vi "数字量输入配置.vi"() -> ()   [LabVIEW 2010] (continued)
              n1455 = local write "单选_第47路"(w57) -> ()
              n1456 = local write "单选_第48路"(w57) -> ()
              n1457 = local write "单选_第49路"(w57) -> ()
              n1458 = local write "单选_第50路"(w57) -> ()
              n1459 = local write "单选_第51路"(w57) -> ()
              n1460 = local write "单选_第52路"(w57) -> ()
              n1461 = local write "单选_第53路"(w57) -> ()
              n1462 = local write "单选_第54路"(w57) -> ()
              n1463 = local write "单选_第55路"(w57) -> ()
              n1464 = local write "单选_第56路"(w57) -> ()
              n1465 = local write "单选_第57路"(w57) -> ()
              n1466 = local write "单选_第58路"(w57) -> ()
              n1467 = local write "单选_第59路"(w57) -> ()
              n1468 = local write "单选_第60路"(w57) -> ()
              n1469 = local write "单选_第61路"(w57) -> ()
              n1470 = local write "单选_第62路"(w57) -> ()
              n1471 = local write "单选_第63路"(w57) -> ()
              n1472 = local write "单选_第64路"(w57) -> ()
              n1473 = local write "单选_第71路"(w57) -> ()
              n1474 = local write "单选_第79路"(w57) -> ()
              n1475 = local write "单选_第65路"(w57) -> ()
              n1476 = local write "单选_第66路"(w57) -> ()
              n1477 = local write "单选_第67路"(w57) -> ()
              n1478 = local write "单选_第68路"(w57) -> ()
              n1479 = local write "单选_第69路"(w57) -> ()
              n1480 = local write "单选_第70路"(w57) -> ()
              n1481 = local write "单选_第72路"(w57) -> ()
              n1482 = local write "单选_第73路"(w57) -> ()
              n1483 = local write "单选_第74路"(w57) -> ()
              n1484 = local write "单选_第75路"(w57) -> ()
              n1485 = local write "单选_第76路"(w57) -> ()
              n1486 = local write "单选_第77路"(w57) -> ()
              n1487 = local write "单选_第78路"(w57) -> ()
              n1488 = local write "单选_第80路"(w57) -> ()
            }
            frame 13 {
              w58 = TRUE
              w59 = FALSE ("单选_第41路")
              n1489 = local write "单选_第1路"(w58) -> ()
              n1490 = local write "单选_第2路"(w58) -> ()
              n1491 = local write "单选_第3路"(w58) -> ()
              n1492 = local write "单选_第4路"(w58) -> ()
              n1493 = local write "单选_第5路"(w58) -> ()
              n1494 = local write "单选_第6路"(w58) -> ()
              n1495 = local write "单选_第7路"(w58) -> ()
              n1496 = local write "单选_第8路"(w58) -> ()
              n1497 = local write "单选_第9路"(w58) -> ()
              n1498 = local write "单选_第10路"(w58) -> ()
              n1499 = local write "单选_第11路"(w58) -> ()
              n1500 = local write "单选_第12路"(w58) -> ()
              n1501 = local write "单选_第13路"(w58) -> ()
              n1502 = local write "单选_第14路"(w59) -> ()
              n1503 = local write "单选_第15路"(w59) -> ()
              n1504 = local write "单选_第16路"(w59) -> ()
              n1505 = local write "单选_第17路"(w59) -> ()
              n1506 = local write "单选_第18路"(w59) -> ()
              n1507 = local write "单选_第19路"(w59) -> ()
              n1508 = local write "单选_第20路"(w59) -> ()
              n1509 = local write "单选_第21路"(w59) -> ()
              n1510 = local write "单选_第22路"(w59) -> ()
              n1511 = local write "单选_第23路"(w59) -> ()
              n1512 = local write "单选_第24路"(w59) -> ()
              n1513 = local write "单选_第25路"(w59) -> ()
              n1514 = local write "单选_第26路"(w59) -> ()
              n1515 = local write "单选_第27路"(w59) -> ()
              n1516 = local write "单选_第28路"(w59) -> ()
              n1517 = local write "单选_第29路"(w59) -> ()
              n1518 = local write "单选_第30路"(w59) -> ()
              n1519 = local write "单选_第31路"(w59) -> ()
              n1520 = local write "单选_第32路"(w59) -> ()
              n1521 = local write "单选_第33路"(w59) -> ()
              n1522 = local write "单选_第34路"(w59) -> ()
              n1523 = local write "单选_第35路"(w59) -> ()
              n1524 = local write "单选_第36路"(w59) -> ()
              n1525 = local write "单选_第37路"(w59) -> ()
              n1526 = local write "单选_第38路"(w59) -> ()
              n1527 = local write "单选_第39路"(w59) -> ()
              n1528 = local write "单选_第40路"(w59) -> ()
              n1529 = local write "单选_第41路"(w59) -> ()
              n1530 = local write "单选_第42路"(w59) -> ()
              n1531 = local write "单选_第43路"(w59) -> ()
              n1532 = local write "单选_第44路"(w59) -> ()
              n1533 = local write "单选_第45路"(w59) -> ()
              n1534 = local write "单选_第46路"(w59) -> ()
              n1535 = local write "单选_第47路"(w59) -> ()
              n1536 = local write "单选_第48路"(w59) -> ()
              n1537 = local write "单选_第49路"(w59) -> ()
              n1538 = local write "单选_第50路"(w59) -> ()
              n1539 = local write "单选_第51路"(w59) -> ()
              n1540 = local write "单选_第52路"(w59) -> ()
              n1541 = local write "单选_第53路"(w59) -> ()
              n1542 = local write "单选_第54路"(w59) -> ()
              n1543 = local write "单选_第55路"(w59) -> ()
              n1544 = local write "单选_第56路"(w59) -> ()
              n1545 = local write "单选_第57路"(w59) -> ()
              n1546 = local write "单选_第58路"(w59) -> ()
              n1547 = local write "单选_第59路"(w59) -> ()
              n1548 = local write "单选_第60路"(w59) -> ()
              n1549 = local write "单选_第61路"(w59) -> ()
              n1550 = local write "单选_第62路"(w59) -> ()
              n1551 = local write "单选_第63路"(w59) -> ()
              n1552 = local write "单选_第64路"(w59) -> ()
              n1553 = local write "单选_第71路"(w59) -> ()
              n1554 = local write "单选_第79路"(w59) -> ()
              n1555 = local write "单选_第65路"(w59) -> ()
              n1556 = local write "单选_第66路"(w59) -> ()
              n1557 = local write "单选_第67路"(w59) -> ()
              n1558 = local write "单选_第68路"(w59) -> ()
              n1559 = local write "单选_第69路"(w59) -> ()
              n1560 = local write "单选_第70路"(w59) -> ()
              n1561 = local write "单选_第72路"(w59) -> ()
              n1562 = local write "单选_第73路"(w59) -> ()
              n1563 = local write "单选_第74路"(w59) -> ()
              n1564 = local write "单选_第75路"(w59) -> ()
              n1565 = local write "单选_第76路"(w59) -> ()
              n1566 = local write "单选_第77路"(w59) -> ()
              n1567 = local write "单选_第78路"(w59) -> ()
              n1568 = local write "单选_第80路"(w59) -> ()
            }
            frame 14 {
              w60 = TRUE
              w61 = FALSE ("单选_第41路")
              n1569 = local write "单选_第1路"(w60) -> ()
              n1570 = local write "单选_第2路"(w60) -> ()
              n1571 = local write "单选_第3路"(w60) -> ()
              n1572 = local write "单选_第4路"(w60) -> ()
              n1573 = local write "单选_第5路"(w60) -> ()
              n1574 = local write "单选_第6路"(w60) -> ()
              n1575 = local write "单选_第7路"(w60) -> ()
              n1576 = local write "单选_第8路"(w60) -> ()
              n1577 = local write "单选_第9路"(w60) -> ()
              n1578 = local write "单选_第10路"(w60) -> ()
              n1579 = local write "单选_第11路"(w60) -> ()
              n1580 = local write "单选_第12路"(w60) -> ()
              n1581 = local write "单选_第13路"(w60) -> ()
              n1582 = local write "单选_第14路"(w60) -> ()
              n1583 = local write "单选_第15路"(w61) -> ()
              n1584 = local write "单选_第16路"(w61) -> ()
              n1585 = local write "单选_第17路"(w61) -> ()
              n1586 = local write "单选_第18路"(w61) -> ()
              n1587 = local write "单选_第19路"(w61) -> ()
              n1588 = local write "单选_第20路"(w61) -> ()
              n1589 = local write "单选_第21路"(w61) -> ()
              n1590 = local write "单选_第22路"(w61) -> ()
              n1591 = local write "单选_第23路"(w61) -> ()
              n1592 = local write "单选_第24路"(w61) -> ()
              n1593 = local write "单选_第25路"(w61) -> ()
              n1594 = local write "单选_第26路"(w61) -> ()
              n1595 = local write "单选_第27路"(w61) -> ()
              n1596 = local write "单选_第28路"(w61) -> ()
              n1597 = local write "单选_第29路"(w61) -> ()
              n1598 = local write "单选_第30路"(w61) -> ()
              n1599 = local write "单选_第31路"(w61) -> ()
              n1600 = local write "单选_第32路"(w61) -> ()
              n1601 = local write "单选_第33路"(w61) -> ()
              n1602 = local write "单选_第34路"(w61) -> ()
              n1603 = local write "单选_第35路"(w61) -> ()
              n1604 = local write "单选_第36路"(w61) -> ()
              n1605 = local write "单选_第37路"(w61) -> ()
              n1606 = local write "单选_第38路"(w61) -> ()
              n1607 = local write "单选_第39路"(w61) -> ()
              n1608 = local write "单选_第40路"(w61) -> ()
              n1609 = local write "单选_第41路"(w61) -> ()
              n1610 = local write "单选_第42路"(w61) -> ()
              n1611 = local write "单选_第43路"(w61) -> ()
              n1612 = local write "单选_第44路"(w61) -> ()
              n1613 = local write "单选_第45路"(w61) -> ()
              n1614 = local write "单选_第46路"(w61) -> ()
              n1615 = local write "单选_第47路"(w61) -> ()
              n1616 = local write "单选_第48路"(w61) -> ()
              n1617 = local write "单选_第49路"(w61) -> ()
              n1618 = local write "单选_第50路"(w61) -> ()
              n1619 = local write "单选_第51路"(w61) -> ()
              n1620 = local write "单选_第52路"(w61) -> ()
              n1621 = local write "单选_第53路"(w61) -> ()
              n1622 = local write "单选_第54路"(w61) -> ()
              n1623 = local write "单选_第55路"(w61) -> ()
              n1624 = local write "单选_第56路"(w61) -> ()
              n1625 = local write "单选_第57路"(w61) -> ()
              n1626 = local write "单选_第58路"(w61) -> ()
              n1627 = local write "单选_第59路"(w61) -> ()
              n1628 = local write "单选_第60路"(w61) -> ()
              n1629 = local write "单选_第61路"(w61) -> ()
              n1630 = local write "单选_第62路"(w61) -> ()
              n1631 = local write "单选_第63路"(w61) -> ()
              n1632 = local write "单选_第64路"(w61) -> ()
              n1633 = local write "单选_第71路"(w61) -> ()
              n1634 = local write "单选_第79路"(w61) -> ()
              n1635 = local write "单选_第65路"(w61) -> ()
              n1636 = local write "单选_第66路"(w61) -> ()
              n1637 = local write "单选_第67路"(w61) -> ()
              n1638 = local write "单选_第68路"(w61) -> ()
              n1639 = local write "单选_第69路"(w61) -> ()
              n1640 = local write "单选_第70路"(w61) -> ()
              n1641 = local write "单选_第72路"(w61) -> ()
              n1642 = local write "单选_第73路"(w61) -> ()
              n1643 = local write "单选_第74路"(w61) -> ()
              n1644 = local write "单选_第75路"(w61) -> ()
              n1645 = local write "单选_第76路"(w61) -> ()
              n1646 = local write "单选_第77路"(w61) -> ()
              n1647 = local write "单选_第78路"(w61) -> ()
              n1648 = local write "单选_第80路"(w61) -> ()
            }
            frame 15 {
              w62 = TRUE
              w63 = FALSE ("单选_第41路")
              n1649 = local write "单选_第1路"(w62) -> ()
              n1650 = local write "单选_第2路"(w62) -> ()
              n1651 = local write "单选_第3路"(w62) -> ()
              n1652 = local write "单选_第4路"(w62) -> ()
              n1653 = local write "单选_第5路"(w62) -> ()
              n1654 = local write "单选_第6路"(w62) -> ()
              n1655 = local write "单选_第7路"(w62) -> ()
              n1656 = local write "单选_第8路"(w62) -> ()
              n1657 = local write "单选_第9路"(w62) -> ()
              n1658 = local write "单选_第10路"(w62) -> ()
              n1659 = local write "单选_第11路"(w62) -> ()
              n1660 = local write "单选_第12路"(w62) -> ()
              n1661 = local write "单选_第13路"(w62) -> ()
              n1662 = local write "单选_第14路"(w62) -> ()
              n1663 = local write "单选_第15路"(w62) -> ()
              n1664 = local write "单选_第16路"(w63) -> ()
              n1665 = local write "单选_第17路"(w63) -> ()
              n1666 = local write "单选_第18路"(w63) -> ()
              n1667 = local write "单选_第19路"(w63) -> ()
              n1668 = local write "单选_第20路"(w63) -> ()
              n1669 = local write "单选_第21路"(w63) -> ()
              n1670 = local write "单选_第22路"(w63) -> ()
              n1671 = local write "单选_第23路"(w63) -> ()
              n1672 = local write "单选_第24路"(w63) -> ()
              n1673 = local write "单选_第25路"(w63) -> ()
              n1674 = local write "单选_第26路"(w63) -> ()
              n1675 = local write "单选_第27路"(w63) -> ()
              n1676 = local write "单选_第28路"(w63) -> ()
              n1677 = local write "单选_第29路"(w63) -> ()
              n1678 = local write "单选_第30路"(w63) -> ()
              n1679 = local write "单选_第31路"(w63) -> ()
              n1680 = local write "单选_第32路"(w63) -> ()
              n1681 = local write "单选_第33路"(w63) -> ()
              n1682 = local write "单选_第34路"(w63) -> ()
              n1683 = local write "单选_第35路"(w63) -> ()
              n1684 = local write "单选_第36路"(w63) -> ()
              n1685 = local write "单选_第37路"(w63) -> ()
              n1686 = local write "单选_第38路"(w63) -> ()
              n1687 = local write "单选_第39路"(w63) -> ()
              n1688 = local write "单选_第40路"(w63) -> ()
              n1689 = local write "单选_第41路"(w63) -> ()
              n1690 = local write "单选_第42路"(w63) -> ()
              n1691 = local write "单选_第43路"(w63) -> ()
              n1692 = local write "单选_第44路"(w63) -> ()
              n1693 = local write "单选_第45路"(w63) -> ()
              n1694 = local write "单选_第46路"(w63) -> ()
              n1695 = local write "单选_第47路"(w63) -> ()
              n1696 = local write "单选_第48路"(w63) -> ()
              n1697 = local write "单选_第49路"(w63) -> ()
              n1698 = local write "单选_第50路"(w63) -> ()
              n1699 = local write "单选_第51路"(w63) -> ()
              n1700 = local write "单选_第52路"(w63) -> ()
              n1701 = local write "单选_第53路"(w63) -> ()
              n1702 = local write "单选_第54路"(w63) -> ()
              n1703 = local write "单选_第55路"(w63) -> ()
              n1704 = local write "单选_第56路"(w63) -> ()
              n1705 = local write "单选_第57路"(w63) -> ()
              n1706 = local write "单选_第58路"(w63) -> ()
              n1707 = local write "单选_第59路"(w63) -> ()
              n1708 = local write "单选_第60路"(w63) -> ()
              n1709 = local write "单选_第61路"(w63) -> ()
              n1710 = local write "单选_第62路"(w63) -> ()
              n1711 = local write "单选_第63路"(w63) -> ()
              n1712 = local write "单选_第64路"(w63) -> ()
              n1713 = local write "单选_第71路"(w63) -> ()
              n1714 = local write "单选_第79路"(w63) -> ()
              n1715 = local write "单选_第65路"(w63) -> ()
              n1716 = local write "单选_第66路"(w63) -> ()
              n1717 = local write "单选_第67路"(w63) -> ()
              n1718 = local write "单选_第68路"(w63) -> ()
              n1719 = local write "单选_第69路"(w63) -> ()
              n1720 = local write "单选_第70路"(w63) -> ()
              n1721 = local write "单选_第72路"(w63) -> ()
              n1722 = local write "单选_第73路"(w63) -> ()
              n1723 = local write "单选_第74路"(w63) -> ()
              n1724 = local write "单选_第75路"(w63) -> ()
              n1725 = local write "单选_第76路"(w63) -> ()
              n1726 = local write "单选_第77路"(w63) -> ()
              n1727 = local write "单选_第78路"(w63) -> ()
              n1728 = local write "单选_第80路"(w63) -> ()
            }
            frame 16 {
              w64 = TRUE
              w65 = FALSE ("单选_第41路")
              n1729 = local write "单选_第1路"(w64) -> ()
              n1730 = local write "单选_第2路"(w64) -> ()
              n1731 = local write "单选_第3路"(w64) -> ()
              n1732 = local write "单选_第4路"(w64) -> ()
              n1733 = local write "单选_第5路"(w64) -> ()
              n1734 = local write "单选_第6路"(w64) -> ()
              n1735 = local write "单选_第7路"(w64) -> ()
              n1736 = local write "单选_第8路"(w64) -> ()
              n1737 = local write "单选_第9路"(w64) -> ()
              n1738 = local write "单选_第10路"(w64) -> ()
              n1739 = local write "单选_第11路"(w64) -> ()
              n1740 = local write "单选_第12路"(w64) -> ()
              n1741 = local write "单选_第13路"(w64) -> ()
              n1742 = local write "单选_第14路"(w64) -> ()
              n1743 = local write "单选_第15路"(w64) -> ()
              n1744 = local write "单选_第16路"(w64) -> ()
              n1745 = local write "单选_第17路"(w65) -> ()
              n1746 = local write "单选_第18路"(w65) -> ()
              n1747 = local write "单选_第19路"(w65) -> ()
              n1748 = local write "单选_第20路"(w65) -> ()
              n1749 = local write "单选_第21路"(w65) -> ()
              n1750 = local write "单选_第22路"(w65) -> ()
              n1751 = local write "单选_第23路"(w65) -> ()
              n1752 = local write "单选_第24路"(w65) -> ()
              n1753 = local write "单选_第25路"(w65) -> ()
              n1754 = local write "单选_第26路"(w65) -> ()
              n1755 = local write "单选_第27路"(w65) -> ()
              n1756 = local write "单选_第28路"(w65) -> ()
              n1757 = local write "单选_第29路"(w65) -> ()
              n1758 = local write "单选_第30路"(w65) -> ()
              n1759 = local write "单选_第31路"(w65) -> ()
              n1760 = local write "单选_第32路"(w65) -> ()
              n1761 = local write "单选_第33路"(w65) -> ()
              n1762 = local write "单选_第34路"(w65) -> ()
              n1763 = local write "单选_第35路"(w65) -> ()
              n1764 = local write "单选_第36路"(w65) -> ()
              n1765 = local write "单选_第37路"(w65) -> ()
              n1766 = local write "单选_第38路"(w65) -> ()
              n1767 = local write "单选_第39路"(w65) -> ()
              n1768 = local write "单选_第40路"(w65) -> ()
              n1769 = local write "单选_第41路"(w65) -> ()
              n1770 = local write "单选_第42路"(w65) -> ()
              n1771 = local write "单选_第43路"(w65) -> ()
              n1772 = local write "单选_第44路"(w65) -> ()
              n1773 = local write "单选_第45路"(w65) -> ()
              n1774 = local write "单选_第46路"(w65) -> ()
              n1775 = local write "单选_第47路"(w65) -> ()
              n1776 = local write "单选_第48路"(w65) -> ()
              n1777 = local write "单选_第49路"(w65) -> ()
              n1778 = local write "单选_第50路"(w65) -> ()
              n1779 = local write "单选_第51路"(w65) -> ()
              n1780 = local write "单选_第52路"(w65) -> ()
              n1781 = local write "单选_第53路"(w65) -> ()
              n1782 = local write "单选_第54路"(w65) -> ()
              n1783 = local write "单选_第55路"(w65) -> ()
              n1784 = local write "单选_第56路"(w65) -> ()
              n1785 = local write "单选_第57路"(w65) -> ()
              n1786 = local write "单选_第58路"(w65) -> ()
              n1787 = local write "单选_第59路"(w65) -> ()
              n1788 = local write "单选_第60路"(w65) -> ()
              n1789 = local write "单选_第61路"(w65) -> ()
              n1790 = local write "单选_第62路"(w65) -> ()
              n1791 = local write "单选_第63路"(w65) -> ()
              n1792 = local write "单选_第64路"(w65) -> ()
              n1793 = local write "单选_第71路"(w65) -> ()
              n1794 = local write "单选_第79路"(w65) -> ()
              n1795 = local write "单选_第65路"(w65) -> ()
              n1796 = local write "单选_第66路"(w65) -> ()
              n1797 = local write "单选_第67路"(w65) -> ()
              n1798 = local write "单选_第68路"(w65) -> ()
              n1799 = local write "单选_第69路"(w65) -> ()
              n1800 = local write "单选_第70路"(w65) -> ()
              n1801 = local write "单选_第72路"(w65) -> ()
              n1802 = local write "单选_第73路"(w65) -> ()
              n1803 = local write "单选_第74路"(w65) -> ()
              n1804 = local write "单选_第75路"(w65) -> ()
              n1805 = local write "单选_第76路"(w65) -> ()
              n1806 = local write "单选_第77路"(w65) -> ()
              n1807 = local write "单选_第78路"(w65) -> ()
              n1808 = local write "单选_第80路"(w65) -> ()
            }
            frame 17 {
              w66 = TRUE
              w67 = FALSE ("单选_第41路")
              n1809 = local write "单选_第1路"(w66) -> ()
              n1810 = local write "单选_第2路"(w66) -> ()
              n1811 = local write "单选_第3路"(w66) -> ()
              n1812 = local write "单选_第4路"(w66) -> ()
              n1813 = local write "单选_第5路"(w66) -> ()
              n1814 = local write "单选_第6路"(w66) -> ()
              n1815 = local write "单选_第7路"(w66) -> ()
              n1816 = local write "单选_第8路"(w66) -> ()
              n1817 = local write "单选_第9路"(w66) -> ()
              n1818 = local write "单选_第10路"(w66) -> ()
              n1819 = local write "单选_第11路"(w66) -> ()
              n1820 = local write "单选_第12路"(w66) -> ()
              n1821 = local write "单选_第13路"(w66) -> ()
              n1822 = local write "单选_第14路"(w66) -> ()
              n1823 = local write "单选_第15路"(w66) -> ()
              n1824 = local write "单选_第16路"(w66) -> ()
              n1825 = local write "单选_第17路"(w66) -> ()
              n1826 = local write "单选_第18路"(w67) -> ()
              n1827 = local write "单选_第19路"(w67) -> ()
              n1828 = local write "单选_第20路"(w67) -> ()
              n1829 = local write "单选_第21路"(w67) -> ()
              n1830 = local write "单选_第22路"(w67) -> ()
              n1831 = local write "单选_第23路"(w67) -> ()
              n1832 = local write "单选_第24路"(w67) -> ()
              n1833 = local write "单选_第25路"(w67) -> ()
              n1834 = local write "单选_第26路"(w67) -> ()
              n1835 = local write "单选_第27路"(w67) -> ()
              n1836 = local write "单选_第28路"(w67) -> ()
              n1837 = local write "单选_第29路"(w67) -> ()
              n1838 = local write "单选_第30路"(w67) -> ()
              n1839 = local write "单选_第31路"(w67) -> ()
              n1840 = local write "单选_第32路"(w67) -> ()
              n1841 = local write "单选_第33路"(w67) -> ()
              n1842 = local write "单选_第34路"(w67) -> ()
              n1843 = local write "单选_第35路"(w67) -> ()
              n1844 = local write "单选_第36路"(w67) -> ()
              n1845 = local write "单选_第37路"(w67) -> ()
              n1846 = local write "单选_第38路"(w67) -> ()
              n1847 = local write "单选_第39路"(w67) -> ()
              n1848 = local write "单选_第40路"(w67) -> ()
              n1849 = local write "单选_第41路"(w67) -> ()
              n1850 = local write "单选_第42路"(w67) -> ()
              n1851 = local write "单选_第43路"(w67) -> ()
              n1852 = local write "单选_第44路"(w67) -> ()
              n1853 = local write "单选_第45路"(w67) -> ()
              n1854 = local write "单选_第46路"(w67) -> ()
              n1855 = local write "单选_第47路"(w67) -> ()
              n1856 = local write "单选_第48路"(w67) -> ()
              n1857 = local write "单选_第49路"(w67) -> ()
              n1858 = local write "单选_第50路"(w67) -> ()
              n1859 = local write "单选_第51路"(w67) -> ()
              n1860 = local write "单选_第52路"(w67) -> ()
              n1861 = local write "单选_第53路"(w67) -> ()
              n1862 = local write "单选_第54路"(w67) -> ()
              n1863 = local write "单选_第55路"(w67) -> ()
              n1864 = local write "单选_第56路"(w67) -> ()
              n1865 = local write "单选_第57路"(w67) -> ()
              n1866 = local write "单选_第58路"(w67) -> ()
              n1867 = local write "单选_第59路"(w67) -> ()
              n1868 = local write "单选_第60路"(w67) -> ()
              n1869 = local write "单选_第61路"(w67) -> ()
              n1870 = local write "单选_第62路"(w67) -> ()
              n1871 = local write "单选_第63路"(w67) -> ()
              n1872 = local write "单选_第64路"(w67) -> ()
              n1873 = local write "单选_第71路"(w67) -> ()
              n1874 = local write "单选_第79路"(w67) -> ()
              n1875 = local write "单选_第65路"(w67) -> ()
              n1876 = local write "单选_第66路"(w67) -> ()
              n1877 = local write "单选_第67路"(w67) -> ()
              n1878 = local write "单选_第68路"(w67) -> ()
              n1879 = local write "单选_第69路"(w67) -> ()
              n1880 = local write "单选_第70路"(w67) -> ()
              n1881 = local write "单选_第72路"(w67) -> ()
              n1882 = local write "单选_第73路"(w67) -> ()
              n1883 = local write "单选_第74路"(w67) -> ()
              n1884 = local write "单选_第75路"(w67) -> ()
              n1885 = local write "单选_第76路"(w67) -> ()
              n1886 = local write "单选_第77路"(w67) -> ()
              n1887 = local write "单选_第78路"(w67) -> ()
              n1888 = local write "单选_第80路"(w67) -> ()
            }
            frame 18 {
              w68 = TRUE
              w69 = FALSE ("单选_第41路")
              n1889 = local write "单选_第1路"(w68) -> ()
              n1890 = local write "单选_第2路"(w68) -> ()
              n1891 = local write "单选_第3路"(w68) -> ()
              n1892 = local write "单选_第4路"(w68) -> ()
              n1893 = local write "单选_第5路"(w68) -> ()
              n1894 = local write "单选_第6路"(w68) -> ()
              n1895 = local write "单选_第7路"(w68) -> ()
              n1896 = local write "单选_第8路"(w68) -> ()
              n1897 = local write "单选_第9路"(w68) -> ()
              n1898 = local write "单选_第10路"(w68) -> ()
              n1899 = local write "单选_第11路"(w68) -> ()
              n1900 = local write "单选_第12路"(w68) -> ()
              n1901 = local write "单选_第13路"(w68) -> ()
              n1902 = local write "单选_第14路"(w68) -> ()
              n1903 = local write "单选_第15路"(w68) -> ()
              n1904 = local write "单选_第16路"(w68) -> ()
              n1905 = local write "单选_第17路"(w68) -> ()
              n1906 = local write "单选_第18路"(w68) -> ()
              n1907 = local write "单选_第19路"(w69) -> ()
              n1908 = local write "单选_第20路"(w69) -> ()
              n1909 = local write "单选_第21路"(w69) -> ()
              n1910 = local write "单选_第22路"(w69) -> ()
              n1911 = local write "单选_第23路"(w69) -> ()
              n1912 = local write "单选_第24路"(w69) -> ()
              n1913 = local write "单选_第25路"(w69) -> ()
              n1914 = local write "单选_第26路"(w69) -> ()
              n1915 = local write "单选_第27路"(w69) -> ()
              n1916 = local write "单选_第28路"(w69) -> ()
              n1917 = local write "单选_第29路"(w69) -> ()
              n1918 = local write "单选_第30路"(w69) -> ()
              n1919 = local write "单选_第31路"(w69) -> ()
              n1920 = local write "单选_第32路"(w69) -> ()
              n1921 = local write "单选_第33路"(w69) -> ()
              n1922 = local write "单选_第34路"(w69) -> ()
              n1923 = local write "单选_第35路"(w69) -> ()
              n1924 = local write "单选_第36路"(w69) -> ()
              n1925 = local write "单选_第37路"(w69) -> ()
              n1926 = local write "单选_第38路"(w69) -> ()
              n1927 = local write "单选_第39路"(w69) -> ()
              n1928 = local write "单选_第40路"(w69) -> ()
              n1929 = local write "单选_第41路"(w69) -> ()
              n1930 = local write "单选_第42路"(w69) -> ()
              n1931 = local write "单选_第43路"(w69) -> ()
              n1932 = local write "单选_第44路"(w69) -> ()
              n1933 = local write "单选_第45路"(w69) -> ()
              n1934 = local write "单选_第46路"(w69) -> ()
              n1935 = local write "单选_第47路"(w69) -> ()
              n1936 = local write "单选_第48路"(w69) -> ()
              n1937 = local write "单选_第49路"(w69) -> ()
              n1938 = local write "单选_第50路"(w69) -> ()
              n1939 = local write "单选_第51路"(w69) -> ()
              n1940 = local write "单选_第52路"(w69) -> ()
              n1941 = local write "单选_第53路"(w69) -> ()
              n1942 = local write "单选_第54路"(w69) -> ()
              n1943 = local write "单选_第55路"(w69) -> ()
              n1944 = local write "单选_第56路"(w69) -> ()
              n1945 = local write "单选_第57路"(w69) -> ()
              n1946 = local write "单选_第58路"(w69) -> ()
              n1947 = local write "单选_第59路"(w69) -> ()
              n1948 = local write "单选_第60路"(w69) -> ()
              n1949 = local write "单选_第61路"(w69) -> ()
              n1950 = local write "单选_第62路"(w69) -> ()
              n1951 = local write "单选_第63路"(w69) -> ()
              n1952 = local write "单选_第64路"(w69) -> ()
              n1953 = local write "单选_第71路"(w69) -> ()
              n1954 = local write "单选_第79路"(w69) -> ()
              n1955 = local write "单选_第65路"(w69) -> ()
              n1956 = local write "单选_第66路"(w69) -> ()
              n1957 = local write "单选_第67路"(w69) -> ()
              n1958 = local write "单选_第68路"(w69) -> ()
              n1959 = local write "单选_第69路"(w69) -> ()
              n1960 = local write "单选_第70路"(w69) -> ()
              n1961 = local write "单选_第72路"(w69) -> ()
              n1962 = local write "单选_第73路"(w69) -> ()
              n1963 = local write "单选_第74路"(w69) -> ()
              n1964 = local write "单选_第75路"(w69) -> ()
              n1965 = local write "单选_第76路"(w69) -> ()
              n1966 = local write "单选_第77路"(w69) -> ()
              n1967 = local write "单选_第78路"(w69) -> ()
              n1968 = local write "单选_第80路"(w69) -> ()
            }
            frame 19 {
              w70 = TRUE
              w71 = FALSE ("单选_第41路")
              n1969 = local write "单选_第1路"(w70) -> ()
              n1970 = local write "单选_第2路"(w70) -> ()
              n1971 = local write "单选_第3路"(w70) -> ()
              n1972 = local write "单选_第4路"(w70) -> ()
              n1973 = local write "单选_第5路"(w70) -> ()
              n1974 = local write "单选_第6路"(w70) -> ()
              n1975 = local write "单选_第7路"(w70) -> ()
              n1976 = local write "单选_第8路"(w70) -> ()
              n1977 = local write "单选_第9路"(w70) -> ()
              n1978 = local write "单选_第10路"(w70) -> ()
              n1979 = local write "单选_第11路"(w70) -> ()
              n1980 = local write "单选_第12路"(w70) -> ()
              n1981 = local write "单选_第13路"(w70) -> ()
              n1982 = local write "单选_第14路"(w70) -> ()
              n1983 = local write "单选_第15路"(w70) -> ()
              n1984 = local write "单选_第16路"(w70) -> ()
              n1985 = local write "单选_第17路"(w70) -> ()
              n1986 = local write "单选_第18路"(w70) -> ()
              n1987 = local write "单选_第19路"(w70) -> ()
              n1988 = local write "单选_第20路"(w71) -> ()
              n1989 = local write "单选_第21路"(w71) -> ()
              n1990 = local write "单选_第22路"(w71) -> ()
              n1991 = local write "单选_第23路"(w71) -> ()
              n1992 = local write "单选_第24路"(w71) -> ()
              n1993 = local write "单选_第25路"(w71) -> ()
              n1994 = local write "单选_第26路"(w71) -> ()
              n1995 = local write "单选_第27路"(w71) -> ()
              n1996 = local write "单选_第28路"(w71) -> ()
              n1997 = local write "单选_第29路"(w71) -> ()
              n1998 = local write "单选_第30路"(w71) -> ()
              n1999 = local write "单选_第31路"(w71) -> ()
              n2000 = local write "单选_第32路"(w71) -> ()
              n2001 = local write "单选_第33路"(w71) -> ()
              n2002 = local write "单选_第34路"(w71) -> ()
              n2003 = local write "单选_第35路"(w71) -> ()
              n2004 = local write "单选_第36路"(w71) -> ()
              n2005 = local write "单选_第37路"(w71) -> ()
              n2006 = local write "单选_第38路"(w71) -> ()
              n2007 = local write "单选_第39路"(w71) -> ()
              n2008 = local write "单选_第40路"(w71) -> ()
              n2009 = local write "单选_第41路"(w71) -> ()
              n2010 = local write "单选_第42路"(w71) -> ()
              n2011 = local write "单选_第43路"(w71) -> ()
              n2012 = local write "单选_第44路"(w71) -> ()
              n2013 = local write "单选_第45路"(w71) -> ()
              n2014 = local write "单选_第46路"(w71) -> ()
              n2015 = local write "单选_第47路"(w71) -> ()
              n2016 = local write "单选_第48路"(w71) -> ()
              n2017 = local write "单选_第49路"(w71) -> ()
              n2018 = local write "单选_第50路"(w71) -> ()
              n2019 = local write "单选_第51路"(w71) -> ()
              n2020 = local write "单选_第52路"(w71) -> ()
              n2021 = local write "单选_第53路"(w71) -> ()
              n2022 = local write "单选_第54路"(w71) -> ()
              n2023 = local write "单选_第55路"(w71) -> ()
              n2024 = local write "单选_第56路"(w71) -> ()
              n2025 = local write "单选_第57路"(w71) -> ()
              n2026 = local write "单选_第58路"(w71) -> ()
              n2027 = local write "单选_第59路"(w71) -> ()
              n2028 = local write "单选_第60路"(w71) -> ()
              n2029 = local write "单选_第61路"(w71) -> ()
              n2030 = local write "单选_第62路"(w71) -> ()
              n2031 = local write "单选_第63路"(w71) -> ()
              n2032 = local write "单选_第64路"(w71) -> ()
              n2033 = local write "单选_第71路"(w71) -> ()
              n2034 = local write "单选_第79路"(w71) -> ()
              n2035 = local write "单选_第65路"(w71) -> ()
              n2036 = local write "单选_第66路"(w71) -> ()
              n2037 = local write "单选_第67路"(w71) -> ()
              n2038 = local write "单选_第68路"(w71) -> ()
              n2039 = local write "单选_第69路"(w71) -> ()
              n2040 = local write "单选_第70路"(w71) -> ()
              n2041 = local write "单选_第72路"(w71) -> ()
              n2042 = local write "单选_第73路"(w71) -> ()
              n2043 = local write "单选_第74路"(w71) -> ()
              n2044 = local write "单选_第75路"(w71) -> ()
              n2045 = local write "单选_第76路"(w71) -> ()
              n2046 = local write "单选_第77路"(w71) -> ()
              n2047 = local write "单选_第78路"(w71) -> ()
              n2048 = local write "单选_第80路"(w71) -> ()
            }
            frame 20 {
              w72 = TRUE
              w73 = FALSE ("单选_第41路")
              n2049 = local write "单选_第1路"(w72) -> ()
              n2050 = local write "单选_第2路"(w72) -> ()
              n2051 = local write "单选_第3路"(w72) -> ()
              n2052 = local write "单选_第4路"(w72) -> ()
              n2053 = local write "单选_第5路"(w72) -> ()
              n2054 = local write "单选_第6路"(w72) -> ()
              n2055 = local write "单选_第7路"(w72) -> ()
              n2056 = local write "单选_第8路"(w72) -> ()
              n2057 = local write "单选_第9路"(w72) -> ()
              n2058 = local write "单选_第10路"(w72) -> ()
              n2059 = local write "单选_第11路"(w72) -> ()
              n2060 = local write "单选_第12路"(w72) -> ()
              n2061 = local write "单选_第13路"(w72) -> ()
              n2062 = local write "单选_第14路"(w72) -> ()
              n2063 = local write "单选_第15路"(w72) -> ()
              n2064 = local write "单选_第16路"(w72) -> ()
              n2065 = local write "单选_第17路"(w72) -> ()
              n2066 = local write "单选_第18路"(w72) -> ()
              n2067 = local write "单选_第19路"(w72) -> ()
              n2068 = local write "单选_第20路"(w72) -> ()
              n2069 = local write "单选_第21路"(w73) -> ()
              n2070 = local write "单选_第22路"(w73) -> ()
              n2071 = local write "单选_第23路"(w73) -> ()
              n2072 = local write "单选_第24路"(w73) -> ()
              n2073 = local write "单选_第25路"(w73) -> ()
              n2074 = local write "单选_第26路"(w73) -> ()
              n2075 = local write "单选_第27路"(w73) -> ()
              n2076 = local write "单选_第28路"(w73) -> ()
              n2077 = local write "单选_第29路"(w73) -> ()
              n2078 = local write "单选_第30路"(w73) -> ()
              n2079 = local write "单选_第31路"(w73) -> ()
              n2080 = local write "单选_第32路"(w73) -> ()
              n2081 = local write "单选_第33路"(w73) -> ()
              n2082 = local write "单选_第34路"(w73) -> ()
              n2083 = local write "单选_第35路"(w73) -> ()
              n2084 = local write "单选_第36路"(w73) -> ()
              n2085 = local write "单选_第37路"(w73) -> ()
              n2086 = local write "单选_第38路"(w73) -> ()
              n2087 = local write "单选_第39路"(w73) -> ()
              n2088 = local write "单选_第40路"(w73) -> ()
              n2089 = local write "单选_第41路"(w73) -> ()
              n2090 = local write "单选_第42路"(w73) -> ()
              n2091 = local write "单选_第43路"(w73) -> ()
              n2092 = local write "单选_第44路"(w73) -> ()
              n2093 = local write "单选_第45路"(w73) -> ()
              n2094 = local write "单选_第46路"(w73) -> ()
              n2095 = local write "单选_第47路"(w73) -> ()
              n2096 = local write "单选_第48路"(w73) -> ()
              n2097 = local write "单选_第49路"(w73) -> ()
              n2098 = local write "单选_第50路"(w73) -> ()
              n2099 = local write "单选_第51路"(w73) -> ()
              n2100 = local write "单选_第52路"(w73) -> ()
              n2101 = local write "单选_第53路"(w73) -> ()
              n2102 = local write "单选_第54路"(w73) -> ()
              n2103 = local write "单选_第55路"(w73) -> ()
              n2104 = local write "单选_第56路"(w73) -> ()
              n2105 = local write "单选_第57路"(w73) -> ()
              n2106 = local write "单选_第58路"(w73) -> ()
              n2107 = local write "单选_第59路"(w73) -> ()
              n2108 = local write "单选_第60路"(w73) -> ()
              n2109 = local write "单选_第61路"(w73) -> ()
              n2110 = local write "单选_第62路"(w73) -> ()
              n2111 = local write "单选_第63路"(w73) -> ()
              n2112 = local write "单选_第64路"(w73) -> ()
              n2113 = local write "单选_第71路"(w73) -> ()
              n2114 = local write "单选_第79路"(w73) -> ()
              n2115 = local write "单选_第65路"(w73) -> ()
              n2116 = local write "单选_第66路"(w73) -> ()
              n2117 = local write "单选_第67路"(w73) -> ()
              n2118 = local write "单选_第68路"(w73) -> ()
              n2119 = local write "单选_第69路"(w73) -> ()
              n2120 = local write "单选_第70路"(w73) -> ()
              n2121 = local write "单选_第72路"(w73) -> ()
              n2122 = local write "单选_第73路"(w73) -> ()
              n2123 = local write "单选_第74路"(w73) -> ()
              n2124 = local write "单选_第75路"(w73) -> ()
              n2125 = local write "单选_第76路"(w73) -> ()
              n2126 = local write "单选_第77路"(w73) -> ()
              n2127 = local write "单选_第78路"(w73) -> ()
              n2128 = local write "单选_第80路"(w73) -> ()
            }
            frame 21 {
              w74 = TRUE
              w75 = FALSE ("单选_第41路")
              n2129 = local write "单选_第1路"(w74) -> ()
              n2130 = local write "单选_第2路"(w74) -> ()
              n2131 = local write "单选_第3路"(w74) -> ()
              n2132 = local write "单选_第4路"(w74) -> ()
              n2133 = local write "单选_第5路"(w74) -> ()
              n2134 = local write "单选_第6路"(w74) -> ()
              n2135 = local write "单选_第7路"(w74) -> ()
              n2136 = local write "单选_第8路"(w74) -> ()
              n2137 = local write "单选_第9路"(w74) -> ()
              n2138 = local write "单选_第10路"(w74) -> ()
              n2139 = local write "单选_第11路"(w74) -> ()
              n2140 = local write "单选_第12路"(w74) -> ()
              n2141 = local write "单选_第13路"(w74) -> ()
              n2142 = local write "单选_第14路"(w74) -> ()
              n2143 = local write "单选_第15路"(w74) -> ()
              n2144 = local write "单选_第16路"(w74) -> ()
              n2145 = local write "单选_第17路"(w74) -> ()
              n2146 = local write "单选_第18路"(w74) -> ()
              n2147 = local write "单选_第19路"(w74) -> ()
              n2148 = local write "单选_第20路"(w74) -> ()
              n2149 = local write "单选_第21路"(w74) -> ()
              n2150 = local write "单选_第22路"(w75) -> ()
              n2151 = local write "单选_第23路"(w75) -> ()
              n2152 = local write "单选_第24路"(w75) -> ()
              n2153 = local write "单选_第25路"(w75) -> ()
              n2154 = local write "单选_第26路"(w75) -> ()
              n2155 = local write "单选_第27路"(w75) -> ()
              n2156 = local write "单选_第28路"(w75) -> ()
              n2157 = local write "单选_第29路"(w75) -> ()
              n2158 = local write "单选_第30路"(w75) -> ()
              n2159 = local write "单选_第31路"(w75) -> ()
              n2160 = local write "单选_第32路"(w75) -> ()
              n2161 = local write "单选_第33路"(w75) -> ()
              n2162 = local write "单选_第34路"(w75) -> ()
              n2163 = local write "单选_第35路"(w75) -> ()
              n2164 = local write "单选_第36路"(w75) -> ()
              n2165 = local write "单选_第37路"(w75) -> ()
              n2166 = local write "单选_第38路"(w75) -> ()
              n2167 = local write "单选_第39路"(w75) -> ()
              n2168 = local write "单选_第40路"(w75) -> ()
              n2169 = local write "单选_第41路"(w75) -> ()
              n2170 = local write "单选_第42路"(w75) -> ()
              n2171 = local write "单选_第43路"(w75) -> ()
              n2172 = local write "单选_第44路"(w75) -> ()
              n2173 = local write "单选_第45路"(w75) -> ()
              n2174 = local write "单选_第46路"(w75) -> ()
              n2175 = local write "单选_第47路"(w75) -> ()
              n2176 = local write "单选_第48路"(w75) -> ()
              n2177 = local write "单选_第49路"(w75) -> ()
              n2178 = local write "单选_第50路"(w75) -> ()
              n2179 = local write "单选_第51路"(w75) -> ()
              n2180 = local write "单选_第52路"(w75) -> ()
              n2181 = local write "单选_第53路"(w75) -> ()
              n2182 = local write "单选_第54路"(w75) -> ()
              n2183 = local write "单选_第55路"(w75) -> ()
              n2184 = local write "单选_第56路"(w75) -> ()
              n2185 = local write "单选_第57路"(w75) -> ()
              n2186 = local write "单选_第58路"(w75) -> ()
              n2187 = local write "单选_第59路"(w75) -> ()
              n2188 = local write "单选_第60路"(w75) -> ()
              n2189 = local write "单选_第61路"(w75) -> ()
              n2190 = local write "单选_第62路"(w75) -> ()
              n2191 = local write "单选_第63路"(w75) -> ()
              n2192 = local write "单选_第64路"(w75) -> ()
              n2193 = local write "单选_第71路"(w75) -> ()
              n2194 = local write "单选_第79路"(w75) -> ()
              n2195 = local write "单选_第65路"(w75) -> ()
              n2196 = local write "单选_第66路"(w75) -> ()
              n2197 = local write "单选_第67路"(w75) -> ()
              n2198 = local write "单选_第68路"(w75) -> ()
              n2199 = local write "单选_第69路"(w75) -> ()
              n2200 = local write "单选_第70路"(w75) -> ()
              n2201 = local write "单选_第72路"(w75) -> ()
              n2202 = local write "单选_第73路"(w75) -> ()
              n2203 = local write "单选_第74路"(w75) -> ()
              n2204 = local write "单选_第75路"(w75) -> ()
              n2205 = local write "单选_第76路"(w75) -> ()
              n2206 = local write "单选_第77路"(w75) -> ()
              n2207 = local write "单选_第78路"(w75) -> ()
              n2208 = local write "单选_第80路"(w75) -> ()
            }
            frame 22 {
              w76 = TRUE
              w77 = FALSE ("单选_第41路")
              n2209 = local write "单选_第1路"(w76) -> ()
              n2210 = local write "单选_第2路"(w76) -> ()
              n2211 = local write "单选_第3路"(w76) -> ()
              n2212 = local write "单选_第4路"(w76) -> ()
              n2213 = local write "单选_第5路"(w76) -> ()
              n2214 = local write "单选_第6路"(w76) -> ()
              n2215 = local write "单选_第7路"(w76) -> ()
              n2216 = local write "单选_第8路"(w76) -> ()
              n2217 = local write "单选_第9路"(w76) -> ()
              n2218 = local write "单选_第10路"(w76) -> ()
              n2219 = local write "单选_第11路"(w76) -> ()
              n2220 = local write "单选_第12路"(w76) -> ()
              n2221 = local write "单选_第13路"(w76) -> ()
              n2222 = local write "单选_第14路"(w76) -> ()
              n2223 = local write "单选_第15路"(w76) -> ()
              n2224 = local write "单选_第16路"(w76) -> ()
              n2225 = local write "单选_第17路"(w76) -> ()
              n2226 = local write "单选_第18路"(w76) -> ()
              n2227 = local write "单选_第19路"(w76) -> ()
              n2228 = local write "单选_第20路"(w76) -> ()
              n2229 = local write "单选_第21路"(w76) -> ()
              n2230 = local write "单选_第22路"(w76) -> ()
              n2231 = local write "单选_第23路"(w77) -> ()
              n2232 = local write "单选_第24路"(w77) -> ()
              n2233 = local write "单选_第25路"(w77) -> ()
              n2234 = local write "单选_第26路"(w77) -> ()
              n2235 = local write "单选_第27路"(w77) -> ()
              n2236 = local write "单选_第28路"(w77) -> ()
              n2237 = local write "单选_第29路"(w77) -> ()
              n2238 = local write "单选_第30路"(w77) -> ()
              n2239 = local write "单选_第31路"(w77) -> ()
              n2240 = local write "单选_第32路"(w77) -> ()
              n2241 = local write "单选_第33路"(w77) -> ()
              n2242 = local write "单选_第34路"(w77) -> ()
              n2243 = local write "单选_第35路"(w77) -> ()
              n2244 = local write "单选_第36路"(w77) -> ()
              n2245 = local write "单选_第37路"(w77) -> ()
              n2246 = local write "单选_第38路"(w77) -> ()
              n2247 = local write "单选_第39路"(w77) -> ()
              n2248 = local write "单选_第40路"(w77) -> ()
              n2249 = local write "单选_第41路"(w77) -> ()
              n2250 = local write "单选_第42路"(w77) -> ()
              n2251 = local write "单选_第43路"(w77) -> ()
              n2252 = local write "单选_第44路"(w77) -> ()
              n2253 = local write "单选_第45路"(w77) -> ()
              n2254 = local write "单选_第46路"(w77) -> ()
              n2255 = local write "单选_第47路"(w77) -> ()
              n2256 = local write "单选_第48路"(w77) -> ()
              n2257 = local write "单选_第49路"(w77) -> ()
              n2258 = local write "单选_第50路"(w77) -> ()
              n2259 = local write "单选_第51路"(w77) -> ()
              n2260 = local write "单选_第52路"(w77) -> ()
              n2261 = local write "单选_第53路"(w77) -> ()
              n2262 = local write "单选_第54路"(w77) -> ()
              n2263 = local write "单选_第55路"(w77) -> ()
              n2264 = local write "单选_第56路"(w77) -> ()
              n2265 = local write "单选_第57路"(w77) -> ()
              n2266 = local write "单选_第58路"(w77) -> ()
              n2267 = local write "单选_第59路"(w77) -> ()
              n2268 = local write "单选_第60路"(w77) -> ()
              n2269 = local write "单选_第61路"(w77) -> ()
              n2270 = local write "单选_第62路"(w77) -> ()
              n2271 = local write "单选_第63路"(w77) -> ()
              n2272 = local write "单选_第64路"(w77) -> ()
              n2273 = local write "单选_第71路"(w77) -> ()
              n2274 = local write "单选_第79路"(w77) -> ()
              n2275 = local write "单选_第65路"(w77) -> ()
              n2276 = local write "单选_第66路"(w77) -> ()
              n2277 = local write "单选_第67路"(w77) -> ()
              n2278 = local write "单选_第68路"(w77) -> ()
              n2279 = local write "单选_第69路"(w77) -> ()
              n2280 = local write "单选_第70路"(w77) -> ()
              n2281 = local write "单选_第72路"(w77) -> ()
              n2282 = local write "单选_第73路"(w77) -> ()
              n2283 = local write "单选_第74路"(w77) -> ()
              n2284 = local write "单选_第75路"(w77) -> ()
              n2285 = local write "单选_第76路"(w77) -> ()
              n2286 = local write "单选_第77路"(w77) -> ()
              n2287 = local write "单选_第78路"(w77) -> ()
              n2288 = local write "单选_第80路"(w77) -> ()
            }
            frame 23 {
              w78 = TRUE
              w79 = FALSE ("单选_第41路")
              n2289 = local write "单选_第1路"(w78) -> ()
              n2290 = local write "单选_第2路"(w78) -> ()
              n2291 = local write "单选_第3路"(w78) -> ()
              n2292 = local write "单选_第4路"(w78) -> ()
              n2293 = local write "单选_第5路"(w78) -> ()
              n2294 = local write "单选_第6路"(w78) -> ()
              n2295 = local write "单选_第7路"(w78) -> ()
              n2296 = local write "单选_第8路"(w78) -> ()
              n2297 = local write "单选_第9路"(w78) -> ()
              n2298 = local write "单选_第10路"(w78) -> ()
              n2299 = local write "单选_第11路"(w78) -> ()
              n2300 = local write "单选_第12路"(w78) -> ()
              n2301 = local write "单选_第13路"(w78) -> ()
              n2302 = local write "单选_第14路"(w78) -> ()
              n2303 = local write "单选_第15路"(w78) -> ()
              n2304 = local write "单选_第16路"(w78) -> ()
              n2305 = local write "单选_第17路"(w78) -> ()
              n2306 = local write "单选_第18路"(w78) -> ()
              n2307 = local write "单选_第19路"(w78) -> ()
              n2308 = local write "单选_第20路"(w78) -> ()
              n2309 = local write "单选_第21路"(w78) -> ()
              n2310 = local write "单选_第22路"(w78) -> ()
              n2311 = local write "单选_第23路"(w78) -> ()
              n2312 = local write "单选_第24路"(w79) -> ()
              n2313 = local write "单选_第25路"(w79) -> ()
              n2314 = local write "单选_第26路"(w79) -> ()
              n2315 = local write "单选_第27路"(w79) -> ()
              n2316 = local write "单选_第28路"(w79) -> ()
              n2317 = local write "单选_第29路"(w79) -> ()
              n2318 = local write "单选_第30路"(w79) -> ()
              n2319 = local write "单选_第31路"(w79) -> ()
              n2320 = local write "单选_第32路"(w79) -> ()
              n2321 = local write "单选_第33路"(w79) -> ()
              n2322 = local write "单选_第34路"(w79) -> ()
              n2323 = local write "单选_第35路"(w79) -> ()
              n2324 = local write "单选_第36路"(w79) -> ()
              n2325 = local write "单选_第37路"(w79) -> ()
              n2326 = local write "单选_第38路"(w79) -> ()
              n2327 = local write "单选_第39路"(w79) -> ()
              n2328 = local write "单选_第40路"(w79) -> ()
              n2329 = local write "单选_第41路"(w79) -> ()
              n2330 = local write "单选_第42路"(w79) -> ()
              n2331 = local write "单选_第43路"(w79) -> ()
              n2332 = local write "单选_第44路"(w79) -> ()
              n2333 = local write "单选_第45路"(w79) -> ()
              n2334 = local write "单选_第46路"(w79) -> ()
              n2335 = local write "单选_第47路"(w79) -> ()
              n2336 = local write "单选_第48路"(w79) -> ()
              n2337 = local write "单选_第49路"(w79) -> ()
              n2338 = local write "单选_第50路"(w79) -> ()
              n2339 = local write "单选_第51路"(w79) -> ()
              n2340 = local write "单选_第52路"(w79) -> ()
              n2341 = local write "单选_第53路"(w79) -> ()
              n2342 = local write "单选_第54路"(w79) -> ()
              n2343 = local write "单选_第55路"(w79) -> ()
              n2344 = local write "单选_第56路"(w79) -> ()
              n2345 = local write "单选_第57路"(w79) -> ()
              n2346 = local write "单选_第58路"(w79) -> ()
              n2347 = local write "单选_第59路"(w79) -> ()
              n2348 = local write "单选_第60路"(w79) -> ()
              n2349 = local write "单选_第61路"(w79) -> ()
              n2350 = local write "单选_第62路"(w79) -> ()
              n2351 = local write "单选_第63路"(w79) -> ()
              n2352 = local write "单选_第64路"(w79) -> ()
              n2353 = local write "单选_第71路"(w79) -> ()
              n2354 = local write "单选_第79路"(w79) -> ()
              n2355 = local write "单选_第65路"(w79) -> ()
              n2356 = local write "单选_第66路"(w79) -> ()
              n2357 = local write "单选_第67路"(w79) -> ()
              n2358 = local write "单选_第68路"(w79) -> ()
              n2359 = local write "单选_第69路"(w79) -> ()
              n2360 = local write "单选_第70路"(w79) -> ()
              n2361 = local write "单选_第72路"(w79) -> ()
              n2362 = local write "单选_第73路"(w79) -> ()
              n2363 = local write "单选_第74路"(w79) -> ()
              n2364 = local write "单选_第75路"(w79) -> ()
              n2365 = local write "单选_第76路"(w79) -> ()
              n2366 = local write "单选_第77路"(w79) -> ()
              n2367 = local write "单选_第78路"(w79) -> ()
              n2368 = local write "单选_第80路"(w79) -> ()
            }
            frame 24 {
              w80 = TRUE
              w81 = FALSE ("单选_第41路")
              n2369 = local write "单选_第1路"(w80) -> ()
              n2370 = local write "单选_第2路"(w80) -> ()
              n2371 = local write "单选_第3路"(w80) -> ()
              n2372 = local write "单选_第4路"(w80) -> ()
              n2373 = local write "单选_第5路"(w80) -> ()
              n2374 = local write "单选_第6路"(w80) -> ()
              n2375 = local write "单选_第7路"(w80) -> ()
              n2376 = local write "单选_第8路"(w80) -> ()
              n2377 = local write "单选_第9路"(w80) -> ()
              n2378 = local write "单选_第10路"(w80) -> ()
              n2379 = local write "单选_第11路"(w80) -> ()
              n2380 = local write "单选_第12路"(w80) -> ()
              n2381 = local write "单选_第13路"(w80) -> ()
              n2382 = local write "单选_第14路"(w80) -> ()
              n2383 = local write "单选_第15路"(w80) -> ()
              n2384 = local write "单选_第16路"(w80) -> ()
              n2385 = local write "单选_第17路"(w80) -> ()
              n2386 = local write "单选_第18路"(w80) -> ()
              n2387 = local write "单选_第19路"(w80) -> ()
              n2388 = local write "单选_第20路"(w80) -> ()
              n2389 = local write "单选_第21路"(w80) -> ()
              n2390 = local write "单选_第22路"(w80) -> ()
              n2391 = local write "单选_第23路"(w80) -> ()
              n2392 = local write "单选_第24路"(w80) -> ()
              n2393 = local write "单选_第25路"(w81) -> ()
              n2394 = local write "单选_第26路"(w81) -> ()
              n2395 = local write "单选_第27路"(w81) -> ()
              n2396 = local write "单选_第28路"(w81) -> ()
              n2397 = local write "单选_第29路"(w81) -> ()
              n2398 = local write "单选_第30路"(w81) -> ()
              n2399 = local write "单选_第31路"(w81) -> ()
              n2400 = local write "单选_第32路"(w81) -> ()
              n2401 = local write "单选_第33路"(w81) -> ()
              n2402 = local write "单选_第34路"(w81) -> ()
              n2403 = local write "单选_第35路"(w81) -> ()
              n2404 = local write "单选_第36路"(w81) -> ()
              n2405 = local write "单选_第37路"(w81) -> ()
              n2406 = local write "单选_第38路"(w81) -> ()
              n2407 = local write "单选_第39路"(w81) -> ()
              n2408 = local write "单选_第40路"(w81) -> ()
              n2409 = local write "单选_第41路"(w81) -> ()
              n2410 = local write "单选_第42路"(w81) -> ()
              n2411 = local write "单选_第43路"(w81) -> ()
              n2412 = local write "单选_第44路"(w81) -> ()
              n2413 = local write "单选_第45路"(w81) -> ()
              n2414 = local write "单选_第46路"(w81) -> ()
              n2415 = local write "单选_第47路"(w81) -> ()
              n2416 = local write "单选_第48路"(w81) -> ()
              n2417 = local write "单选_第49路"(w81) -> ()
              n2418 = local write "单选_第50路"(w81) -> ()
              n2419 = local write "单选_第51路"(w81) -> ()
              n2420 = local write "单选_第52路"(w81) -> ()
              n2421 = local write "单选_第53路"(w81) -> ()
              n2422 = local write "单选_第54路"(w81) -> ()
              n2423 = local write "单选_第55路"(w81) -> ()
              n2424 = local write "单选_第56路"(w81) -> ()
              n2425 = local write "单选_第57路"(w81) -> ()
              n2426 = local write "单选_第58路"(w81) -> ()
              n2427 = local write "单选_第59路"(w81) -> ()
              n2428 = local write "单选_第60路"(w81) -> ()
              n2429 = local write "单选_第61路"(w81) -> ()
              n2430 = local write "单选_第62路"(w81) -> ()
              n2431 = local write "单选_第63路"(w81) -> ()
              n2432 = local write "单选_第64路"(w81) -> ()
              n2433 = local write "单选_第71路"(w81) -> ()
              n2434 = local write "单选_第79路"(w81) -> ()
              n2435 = local write "单选_第65路"(w81) -> ()
              n2436 = local write "单选_第66路"(w81) -> ()
              n2437 = local write "单选_第67路"(w81) -> ()
              n2438 = local write "单选_第68路"(w81) -> ()
              n2439 = local write "单选_第69路"(w81) -> ()
              n2440 = local write "单选_第70路"(w81) -> ()
              n2441 = local write "单选_第72路"(w81) -> ()
              n2442 = local write "单选_第73路"(w81) -> ()
              n2443 = local write "单选_第74路"(w81) -> ()
              n2444 = local write "单选_第75路"(w81) -> ()
              n2445 = local write "单选_第76路"(w81) -> ()
              n2446 = local write "单选_第77路"(w81) -> ()
              n2447 = local write "单选_第78路"(w81) -> ()
              n2448 = local write "单选_第80路"(w81) -> ()
            }
            frame 25 {
              w82 = TRUE
              w83 = FALSE ("单选_第41路")
              n2449 = local write "单选_第1路"(w82) -> ()
              n2450 = local write "单选_第2路"(w82) -> ()
              n2451 = local write "单选_第3路"(w82) -> ()
              n2452 = local write "单选_第4路"(w82) -> ()
              n2453 = local write "单选_第5路"(w82) -> ()
              n2454 = local write "单选_第6路"(w82) -> ()
              n2455 = local write "单选_第7路"(w82) -> ()
              n2456 = local write "单选_第8路"(w82) -> ()
              n2457 = local write "单选_第9路"(w82) -> ()
              n2458 = local write "单选_第10路"(w82) -> ()
              n2459 = local write "单选_第11路"(w82) -> ()
              n2460 = local write "单选_第12路"(w82) -> ()
              n2461 = local write "单选_第13路"(w82) -> ()
              n2462 = local write "单选_第14路"(w82) -> ()
              n2463 = local write "单选_第15路"(w82) -> ()
              n2464 = local write "单选_第16路"(w82) -> ()
